vi "Comparacion_datos_bidireccionalidad.vi"() -> ()   [LabVIEW 2015]
panel:
  out "error out 2":errorcluster
  in  "array 2":path[](array[path])=[path "C:/Users/gfernandez/Google Drive/Labview/W&RD_Euskotren/Host/Prueba/Archivos_necesarios_Procesado_Bidire/Trenesv/0001_2013-06-05_13-06-23_0.bin", path "C:/Users/gfernandez/Google Drive/Labview/W&RD_Euskotren/Host/Prueba/Archivos_necesarios_Procesado_Bidire/Trenesv/0001_2013-06-05_13-06-23_2.bin", path "C:/Users/gfernandez/Google Drive/Labview/W&RD_Euskotren/Host/Prueba/Archivos_necesarios_Procesado_Bidire/Trenesv/0001_2013-06-05_13-06-23_4.bin", path "C:/Users/gfernandez/Google Drive/Labview/W&RD_Euskotren/Host/Prueba/Archivos_necesarios_Procesado_Bidire/Trenesv/0001_2013-06-05_13-06-23_6.bin", path "C:/Users/gfernandez/Google Drive/Labview/W&RD_Euskotren/Host/Prueba/Archivos_necesarios_Procesado_Bidire/Trenesv/0001_2013-06-05_13-06-23_8.bin"]
  out "Max RMS Ruedas":dbl[][](array[numeric])
  out "Distancias generales":dbl[](array[numeric])
  out "Puntos iniciales de las ventanas":dbl[](array[numeric])
  out "Distancia de acelerómetros":dbl[](array[numeric])
  out "error out":errorcluster
  in  "array":path[](array[path])=[path "C:/Users/gfernandez/Google Drive/Labview/W&RD_Euskotren/Host/Prueba/Archivos_necesarios_Procesado_Bidire/Trenesi/0001_2013-06-05_13-06-23_0.bin", path "C:/Users/gfernandez/Google Drive/Labview/W&RD_Euskotren/Host/Prueba/Archivos_necesarios_Procesado_Bidire/Trenesi/0001_2013-06-05_13-06-23_2.bin", path "C:/Users/gfernandez/Google Drive/Labview/W&RD_Euskotren/Host/Prueba/Archivos_necesarios_Procesado_Bidire/Trenesi/0001_2013-06-05_13-06-23_4.bin", path "C:/Users/gfernandez/Google Drive/Labview/W&RD_Euskotren/Host/Prueba/Archivos_necesarios_Procesado_Bidire/Trenesi/0001_2013-06-05_13-06-23_6.bin", path "C:/Users/gfernandez/Google Drive/Labview/W&RD_Euskotren/Host/Prueba/Archivos_necesarios_Procesado_Bidire/Trenesi/0001_2013-06-05_13-06-23_8.bin"]
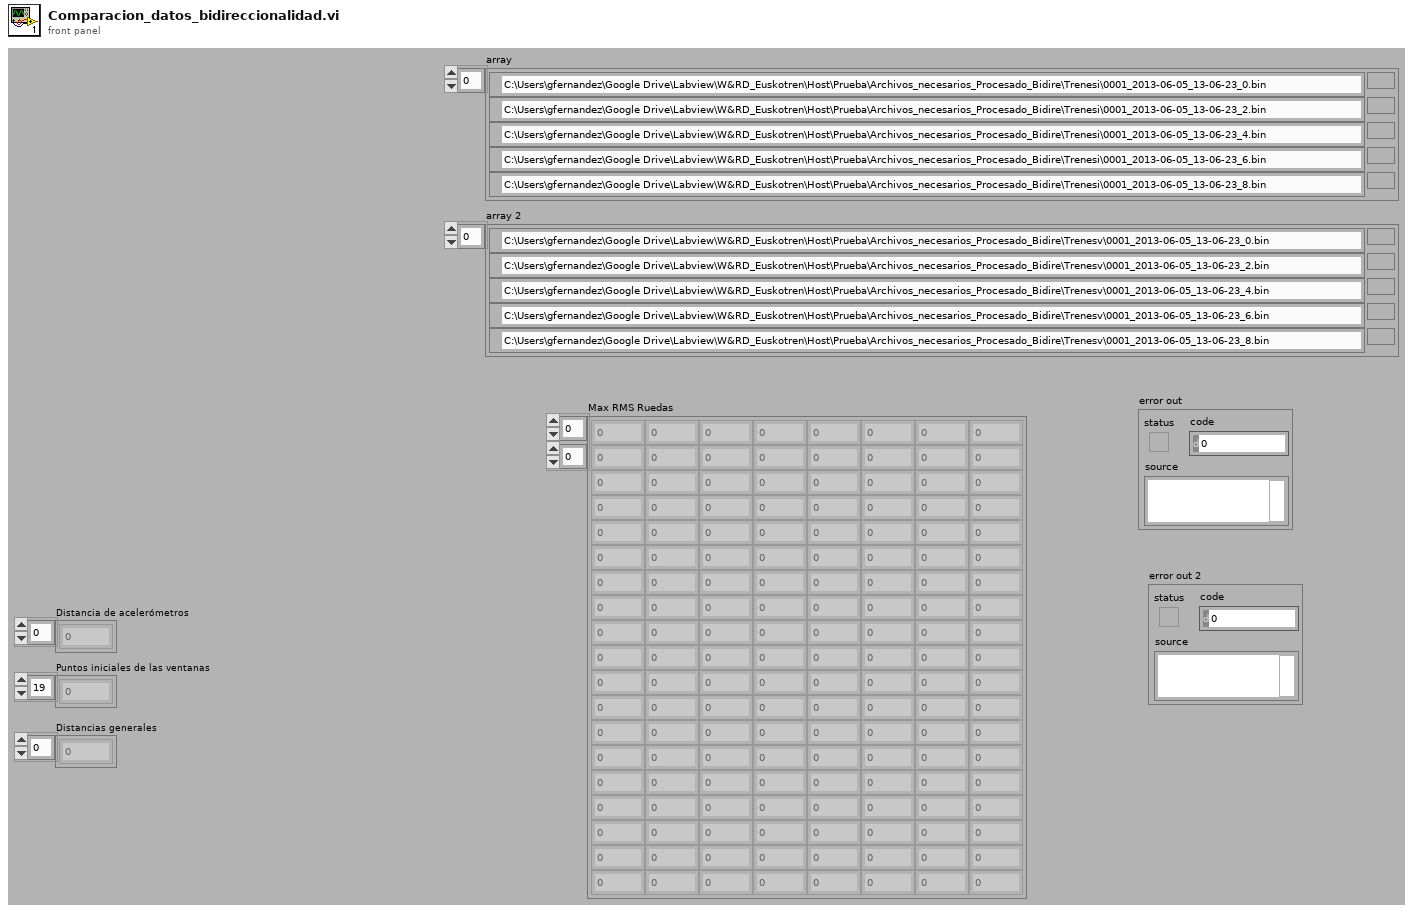
[diagram p1: front panel]
types:
  T1 = enum16{"big-endian, network order", "native, host order", "little-endian"}
  T2 = cluster{"error IO":errorcluster, bool[], u32[], string[], dbl[]}
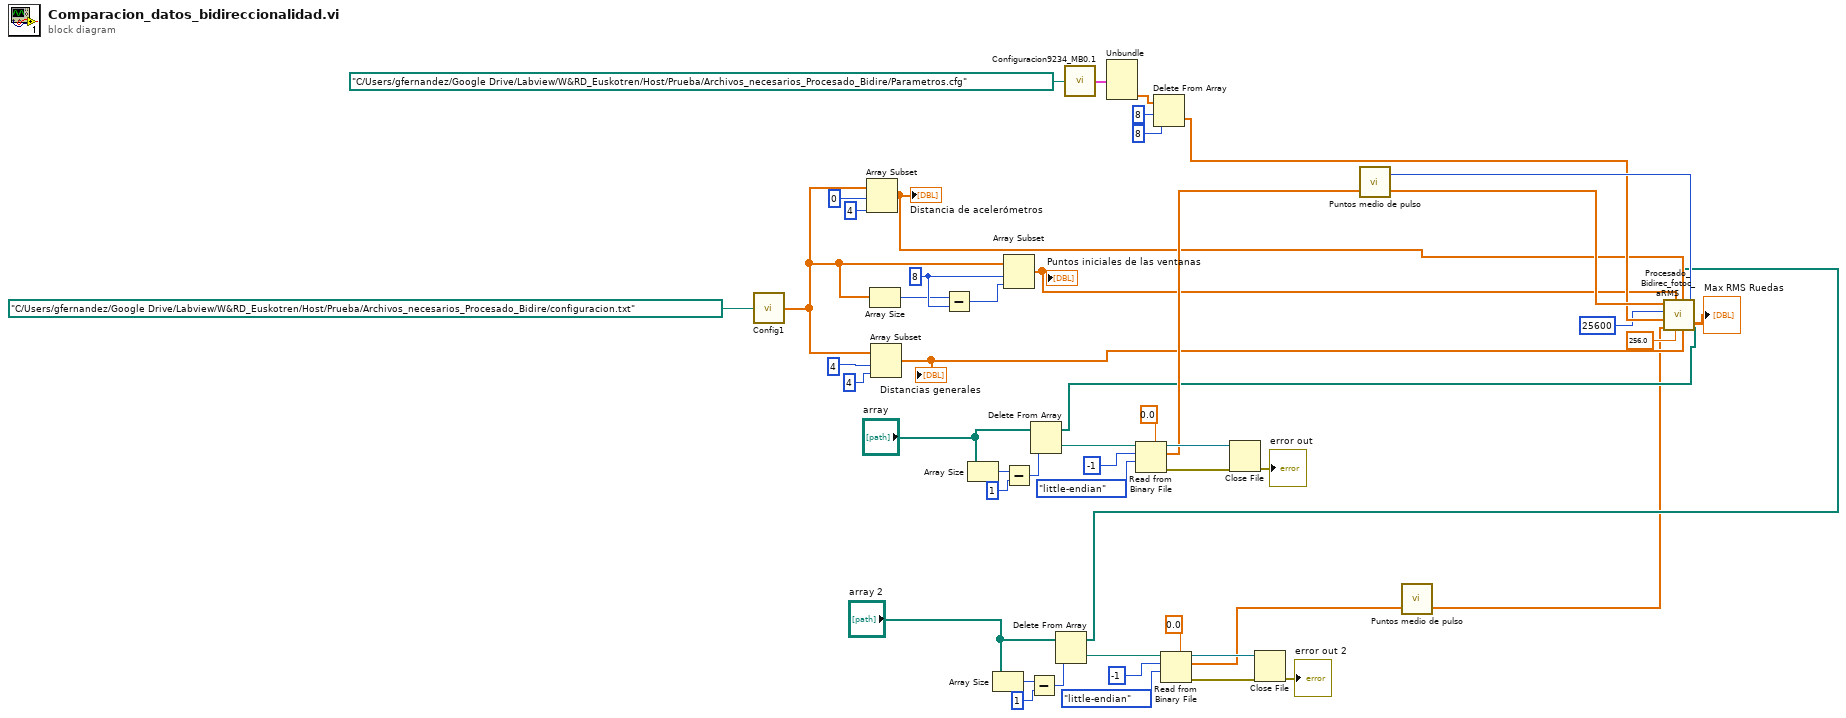
[diagram p0: block diagram]
diagram:
  w22 = 8 ("index")
  n1 = call "Config1.vi"("file path (dialog if empty)"=path "C:/Users/gfernandez/Google Drive/Labview/W&RD_Euskotren/Host/Prueba/Archivos_necesarios_Procesado_Bidire/configuracion.txt") -> ("Distancias"=w20:dbl[])
  n2 = Array Subset(array=w20, index=0, length=4) -> (w18:dbl[])
  "Distancia de acelerómetros" <- w18
  n3 = Array Size(array=w20) -> (size(s)=w21:i32)
  n4 = Array Subset(array=w20, index=4, length=4) -> (w16:dbl[])
  "Distancias generales" <- w16
  n5 = Subtract(x=w21, y=w22) -> (x-y=w23:i32)
  n6 = Array Size(array="array") -> (size(s)=w43:i32)
  n7 = Array Size(array="array 2") -> (size(s)=w12:i32)
  n8 = Array Subset(array=w20, index=w22, length=w23) -> (w17:dbl[])
  "Puntos iniciales de las ventanas" <- w17
  n9 = Subtract(x=w43, y=1 ("length")) -> (x-y=w45:i32)
  n10 = Subtract(x=w12, y=1 ("length")) -> (x-y=w14:i32)
  n11 = Delete From Array(array="array", index=w45) -> (deleted portion=w42:path, array with subset deleted=w29:path[])  [unwired: 1 in]
  n12 = Delete From Array(array="array 2", index=w14) -> (deleted portion=w11:path, array with subset deleted=w3:path[])  [unwired: 1 in]
  n13 = call "Configuracion9234_MB0.1.vi"("configuration file path"=path "C:/Users/gfernandez/Google Drive/Labview/W&RD_Euskotren/Host/Prueba/Archivos_necesarios_Procesado_Bidire/Parametros.cfg" ("file path (dialog if empty)")) -> ("output cluster"=w50:T2)
  n14 = Unbundle(w50) -> (w46:dbl[])  [unwired: 4 out]
  n15 = Read from Binary File(5:sgl 0.0, 9:T1."little-endian" ("byte order (0:big-endian, network order)"), 10:-1 ("count (1)"), 11:w42) -> (0:w40:errorcluster, 2:w35:sgl[], 3:w41:refnum<file>)  [unwired: 1 in, 2 out]
  n16 = Delete From Array(array=w46, length=8, index=8) -> (deleted portion=w31:dbl[])  [unwired: 1 out]
  n17 = Read from Binary File(5:sgl 0.0, 9:T1."little-endian" ("byte order (0:big-endian, network order)"), 10:-1 ("count (1)"), 11:w11) -> (0:w9:errorcluster, 2:w2:sgl[], 3:w10:refnum<file>)  [unwired: 1 in, 2 out]
  n18 = Close File(refnum=w41, error in=w40) -> (error out=→"error out":errorcluster)  [unwired: 1 out]
  n19 = Close File(refnum=w10, error in=w9) -> (error out=→"error out 2":errorcluster)  [unwired: 1 out]
  n20 = call "Puntos medio de pulso.vi"("DI Inductivo"=w35) -> ("Puntos"=w32:sgl[], "Número de ejes"=w33:i32)  [unwired: 1 in]
  n21 = call "Puntos medio de pulso.vi"("DI Inductivo"=w2) -> ("Puntos"=w1:sgl[])  [unwired: 1 in, 1 out]
  n22 = call "Procesado_Bidirec_fotoc_aRMS.vi"("Paths_canales_aRMS"=w29, "Distancias generales (m)"=w16, "Distancias\nacelerometros"=w18, "Ejes Procesados"=w33, "Paths_canales_aRMS 2"=w3, "dt RMS 2"=256.0, "Distancias centrales de las ruedas\n               configuración (m)"=w17, "Puntos 2"=w1, "Parámetros acelerómetros"=w31, "Frecuencia de muestreo"=25600 ("value"), "Puntos"=w32) -> ("Max RMS Ruedas"=→"Max RMS Ruedas":dbl[][])
